vi "Init.vi"(8 "error in":errorcluster, 10 "IConfigure":refnum<class "IConfigure.lvclass">, 11 "Fgen Base in":refnum<class "FGEN Base.lvclass">) -> (0 "error out":errorcluster, 3 "Fgen Base out":refnum<class "FGEN Base.lvclass">)   [LabVIEW 2023, in "FGEN.lvlib" / "FGEN Base.lvlib" / "FGEN Base.lvclass"]
uses:
  FGEN Base.lvclass
  Interfaces/IConfigure/IConfigure.lvclass
  FGEN Base.lvclass/FGEN Base.ctl
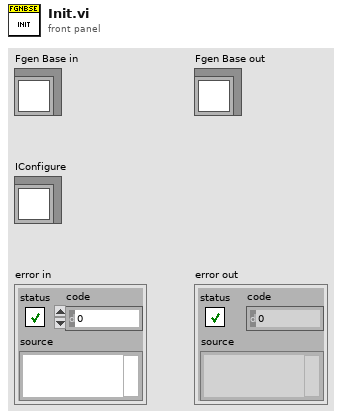
[diagram p1: front panel]
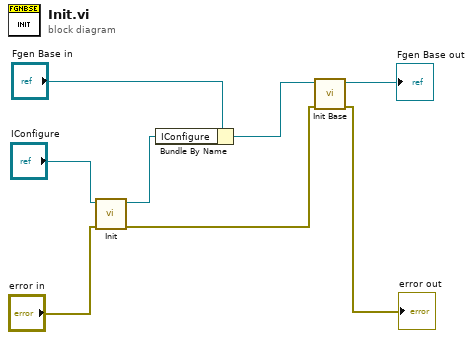
[diagram p0: block diagram]
diagram:
  n1 = call-dynamic "Init.vi"("error in"="error in", "IConfigure in"="IConfigure") -> ("error out"=w7:errorcluster, "IConfigure out"=w8:refnum<class "IConfigure.lvclass">)  [unwired: 8 in]
  n2 = Bundle By Name(cluster="Fgen Base in", "IConfigure"=w8) -> (w6:refnum<class "FGEN Base.lvclass">)
  n3 = call-dynamic "Init Base.vi"("Error In"=w7, "object in"=w6) -> ("Error Out"=→"error out":errorcluster, "object out"=→"Fgen Base out":refnum<class "FGEN Base.lvclass">)  [unwired: 8 in]
